vi "SelMenuFunc.vi"(8 "error in (no error)":errorcluster caption="entrée d'erreur (pas d'erreur)", 11 "AvailFunc":string[](array[string])) -> (0 "error out":errorcluster caption="sortie d'erreur", 1 "Canceled":bool, 2 "Selected Panel":string, 3 "PanelIndex":i32 caption="Available Function Panels")   [LabVIEW 2019, in "BaseDevice.lvclass"]
uses:
  BaseDevice.lvclass
panel:
  in  "Cancel":bool
  in  "Load":bool
  in  "Available Function Panel":u16(ring) caption="Available Menu Panels" items=["Control Panel"]
  # "Select the panel to load for this function"
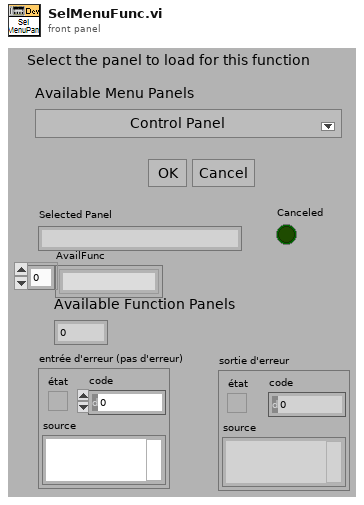
[diagram p1: front panel]
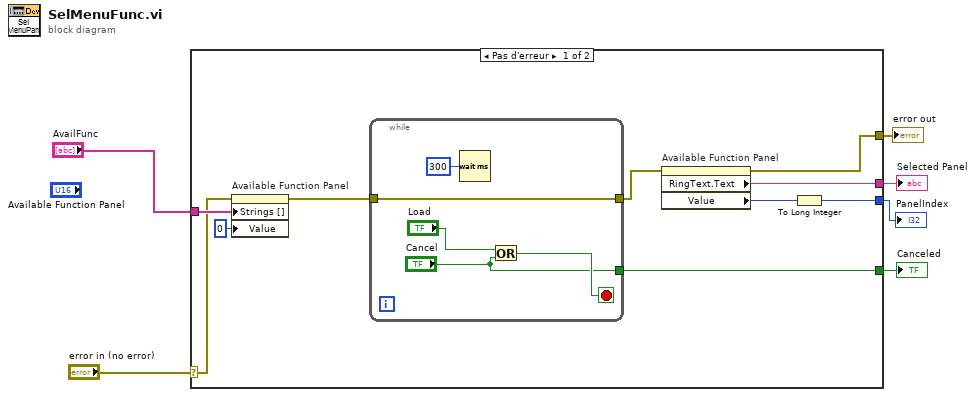
[diagram p0: block diagram]
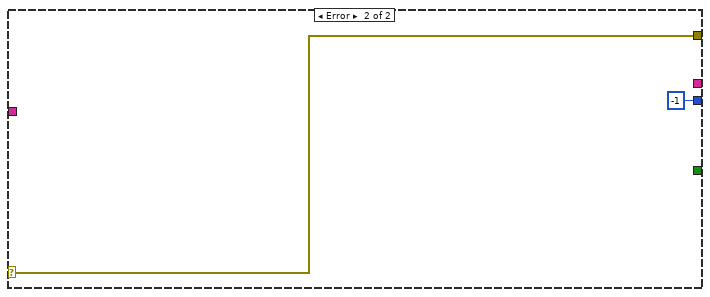
[diagram p2: hidden frame]
diagram:
  n1 = case shown="Pas d'erreur" "error in (no error)" {
    selector: "error in (no error)" -> [w13 w23]
    tunnel: [w10 w23] -> w5
    tunnel: [w16 _] -> w4
    tunnel: "AvailFunc" -> [w14 _]
    tunnel: [w9 _] -> w2
    tunnel: [w7 -1 ("Value")] -> w1
    frame No Error {
      n2 = property on="Available Function Panel" class="MDér (strict)"(error in=w13, "Strings []"=w14, "Value"=u16 0) -> (error out=w12:errorcluster)  [unwired: 1 in, 1 out]
      n3 = while {
        tunnel: ["Cancel"] -> w16
        tunnel: [w18] -> w11
        tunnel: w12 -> [w18]
        stop <- w20 stop-if-true
        n4 = Wait (ms)(milliseconds to wait=u32 300 ("attente (ms)")) -> ()  [unwired: 1 out]
        n5 = Or(x="Load", y="Cancel") -> (x .or. y?=w20:bool)
      }
      n6 = property on="Available Function Panel" class="MDér (strict)"(error in=w11) -> (error out=w10:errorcluster, "RingText.Text"=w9:string, "Value"=w8:u16)  [unwired: 1 in, 1 out]
      n7 = To Long Integer(number=w8) -> (32bit integer=w7:i32)
    }
    frame Error {
    }
  }
  "error out" <- w5
  "Selected Panel" <- w2
  "Canceled" <- w4
  "PanelIndex" <- w1
